vi "Read Marker Values[].vi"(9 "GraphScale in":refnum<class "GraphScale.lvclass">) -> (3 "GraphScale out":refnum<class "GraphScale.lvclass">, 4 "Marker Values[]":dbl[](array[numeric]))   [LabVIEW 2014, in "GraphScale.lvclass"]
uses:
  GraphScale.lvclass
  GraphScale.lvclass/GraphScale.ctl
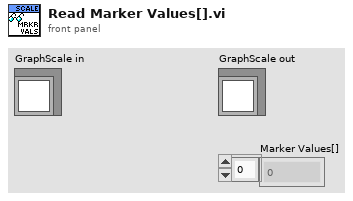
[diagram p1: front panel]
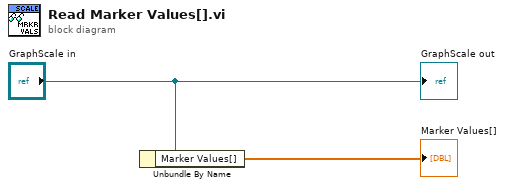
[diagram p0: block diagram]
diagram:
  n1 = Unbundle By Name("GraphScale in") -> ("Marker Values[]"=→"Marker Values[]":dbl[])
  "GraphScale out" <- "GraphScale in"
